vi "Status_check.vi"(8 "错误输入（无错误）":errorcluster, 10 "Status Code":string, 11 "VISA引用句柄输入":refnum<visa-resource-name>) -> (0 "错误输出":errorcluster, 1 "VISA资源名称输出":refnum<visa-resource-name>, 3 "当前电流值":string)   [LabVIEW 2012]
panel:
  out "键盘锁":string="CC"
  out "On/Off":string="CC"
  out "过压":string="CC"
  out "蜂鸣器":string="CC"
  out "测量模式":string="CC"
  out "过温":string="CC"
  out "CC/CV":string="CC"
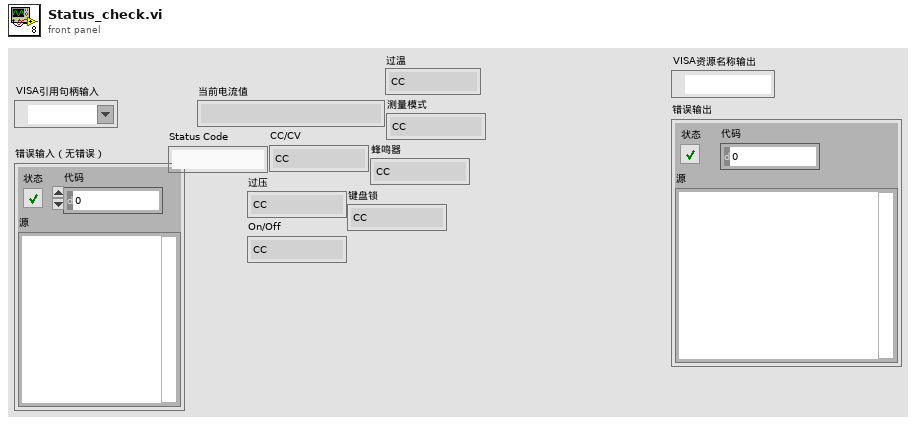
[diagram p1: front panel]
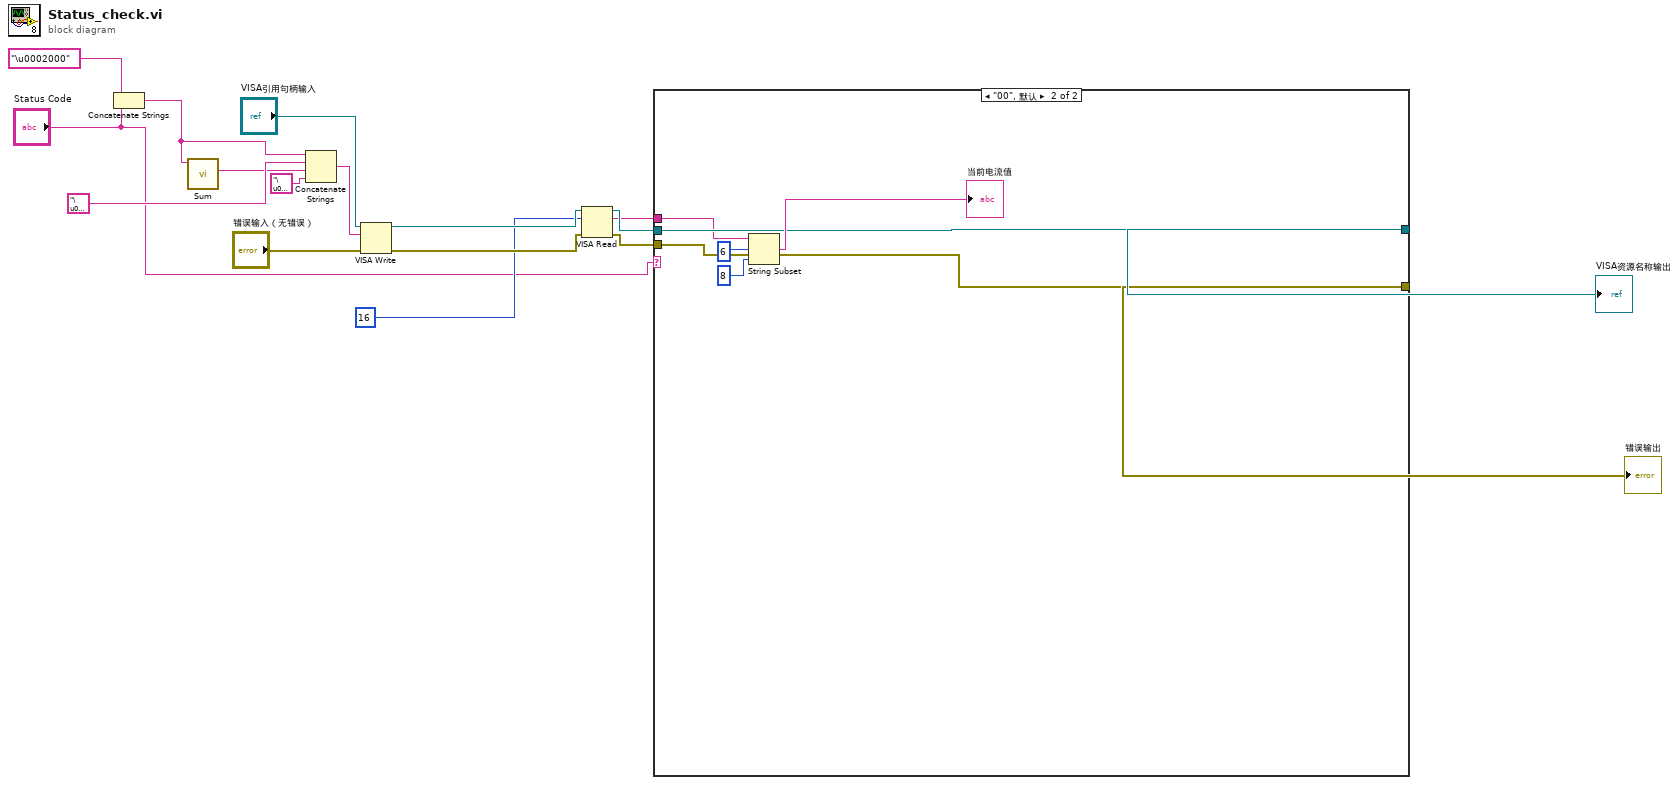
[diagram p0: block diagram]
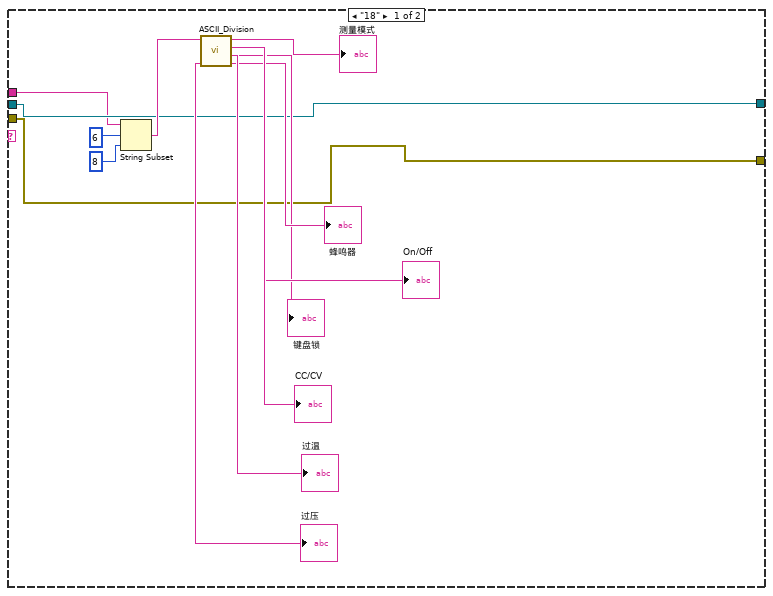
[diagram p2: hidden frame]
diagram:
  n1 = Concatenate Strings("\u0002000", "Status Code") -> (w11:string)
  n2 = call "Sum.vi"("连接的字符串"=w11) -> ("string"=w12:string)  [unwired: 8 in, 2 out]
  n3 = Concatenate Strings(w11, "\u0004", w12, "\u0003") -> (w14:string)
  n4 = VISA Write(VISA resource name="VISA引用句柄输入", write buffer=w14, error in (no error)="错误输入（无错误）") -> (VISA resource name out=w6:refnum<visa-resource-name>, error out=w7:errorcluster)  [unwired: 1 out]
  n5 = VISA Read(VISA resource name=w6, byte count=16, error in (no error)=w7) -> (VISA resource name out=w3:refnum<visa-resource-name>, read buffer=w1:string, error out=w2:errorcluster)  [unwired: 1 out]
  n6 = case shown="\"00\", 默认" "Status Code" {
    tunnel: w3 -> [w20 w33]
    tunnel: [w20 w33] -> w9
    tunnel: [w19 w32] -> w8
    tunnel: w2 -> [w19 w32]
    tunnel: w1 -> [w18 w31]
    frame "18" {
      n7 = String Subset(string=w18, offset (0)=6, length (rest)=8) -> (substring=w28:string)
      n8 = call "ASCII_Division.vi"("字符串"=w28) -> ("蜂鸣器"=→"蜂鸣器":string, "键盘锁"=→"键盘锁":string, "On/Off"=→"On/Off":string, "测量模式"=→"测量模式":string, "过压"=→"过压":string, "过温"=→"过温":string, "CC/CV"=→"CC/CV":string)  [unwired: 4 in]
    }
    frame "00", Default {
      n9 = String Subset(string=w31, offset (0)=6, length (rest)=8) -> (substring=→"当前电流值":string)
    }
  }
  "VISA资源名称输出" <- w9
  "错误输出" <- w8
